vi "append_JSON_data.vi"(0 "JSON in":string="{\"test\":\"hello\"}", 5 "new_key":string="datatype", 7 "new_value":string="float", 11 "error in (no error)":errorcluster) -> (6 "return value":string, 15 "error out":errorcluster)   [LabVIEW 2019, in "mmW_commands.lvlib"]
uses:
  mmW_commands.lvlib
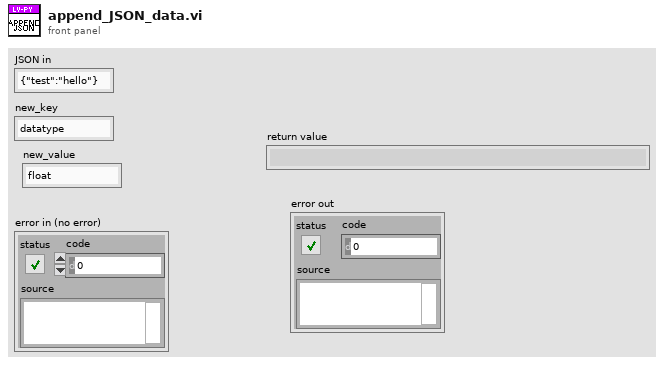
[diagram p1: front panel]
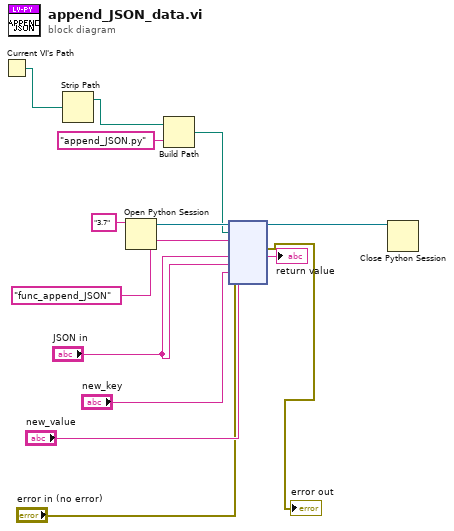
[diagram p0: block diagram]
diagram:
  n1 = Current VI's Path() -> (path=w11:path)
  n2 = Strip Path(path=w11) -> (stripped path=w10:path)  [unwired: 1 out]
  n3 = Open Python Session(python version="3.7" ("Python version")) -> (session out=w13:refnum<k35>)  [unwired: 2 in, 1 out]
  n4 = Build Path(base path=w10, name or relative path="append_JSON.py") -> (appended path=w8:path)
  n5 = node(w13, w8, "func_append_JSON" ("function name"), "error in (no error)", "JSON in", "JSON in", "new_key", "new_value") -> (w12:refnum<k35>, →"error out":errorcluster, →"return value":string)  [unwired: 3 in, 2 out]
  n6 = Close Python Session(session in=w12) -> ()  [unwired: 1 in, 1 out]
